vi "Device in Stack.vi"(8 "error in (no error)":errorcluster, 10 "Device in":refnum<class "Device.lvclass">, 11 "Stack in":refnum<class "Device.lvclass">[](array[class])) -> (0 "error out":errorcluster, 1 "Stack Index":i32, 2 "Device found?":bool, 3 "Stack out":refnum<class "Device.lvclass">[](array[class]))   [LabVIEW 2011, in "Tinkerforge.lvlib" / "Device.lvclass"]
doc: "This VI searches if the given Device is present in the Stack."
uses:
  Device.lvclass
  Device.lvclass/Device.ctl
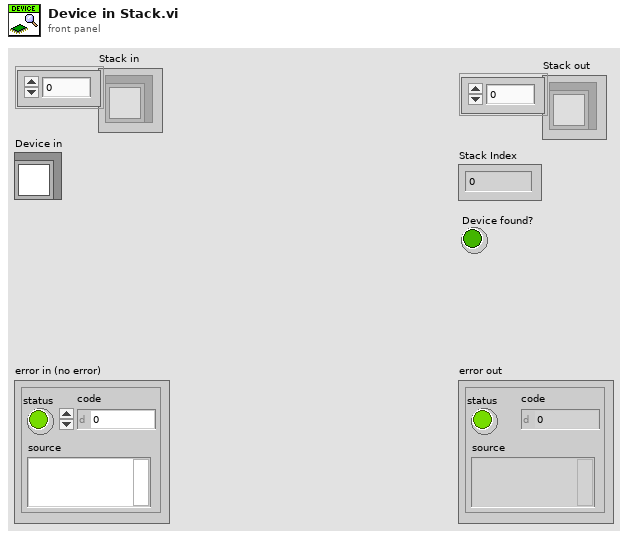
[diagram p1: front panel]
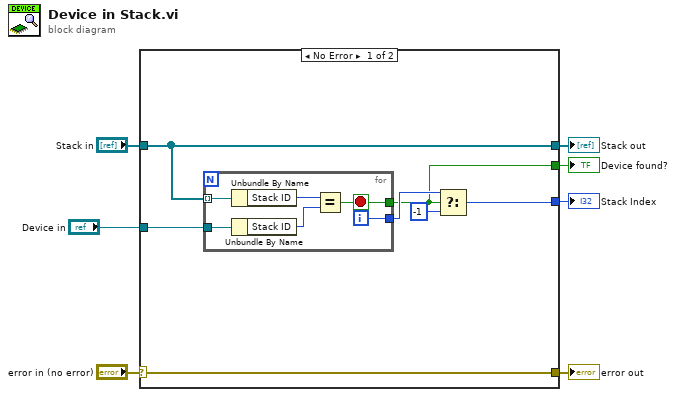
[diagram p0: block diagram]
diagram:
  n1 = case shown="No Error" "error in (no error)" {
    selector: "error in (no error)" -> [w14 w22]
    tunnel: [w14 w22] -> w6
    tunnel: "Stack in" -> [w10 w21]
    tunnel: [w10 w21] -> w4
    tunnel: [w11 _] -> w3
    tunnel: [w9 _] -> w2
    tunnel: "Device in" -> [w8 _]
    frame No Error {
      n2 = for {
        tunnel: w10 -> [w20] mode=indexing
        tunnel: [w18] -> w13
        tunnel: [w17] -> w11
        tunnel: w8 -> [w16]
        i -> [w18]
        stop <- w17 stop-if-true
        n3 = Unbundle By Name(w20) -> ("Stack ID"=w19:u8)
        n4 = Unbundle By Name(w16) -> ("Stack ID"=w15:u8)
        n5 = Equal?(x=w19, y=w15) -> (x = y?=w17:bool)
      }
      n6 = Select(t=w13, s=w11, f=-1) -> (s? t:f=w9:i32)
    }
    frame Error {
    }
  }
  "error out" <- w6
  "Stack out" <- w4
  "Device found?" <- w3
  "Stack Index" <- w2
